vi "helper-RH-create.vi"(7 "Virtual Name":string="_RH", 8 "error in":errorcluster, 9 "record path format OCS\\DB\\%s.* (DISABLE IF EMPTY)":string="OCS\\\\DB\\\\%s.*", 10 "Twet":dbl, 11 "Tdry":dbl) -> (0 "error out":errorcluster, 2 "RH":dbl, 3 "result":string)   [LabVIEW 2024]
uses:
  controls/enumVarCtrlIO.ctl
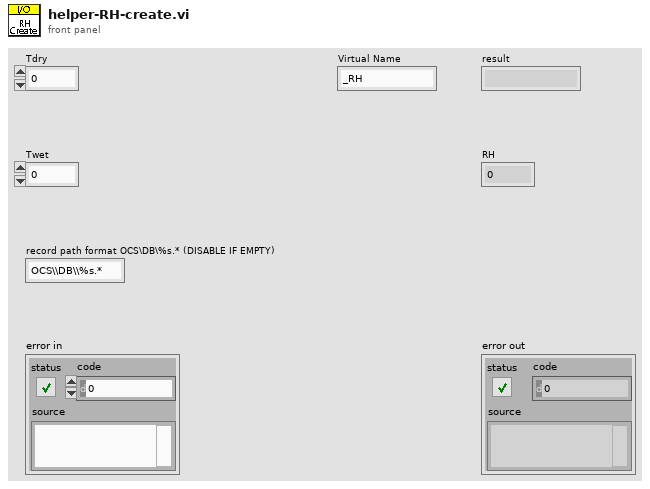
[diagram p1: front panel]
types:
  T1 = typedef "enumVarCtrlIO.ctl" = enum16{"IO Get By Key", "IO List Configs", "IO Add By Key", "IO Modify Value By Key", "IO Modify Calib By Key", "IO Modify ADDR By Key", "IO Modify Mode By Key", "IO Modify Type By Key", "IO Modify Name By Key", "IO Remove By Key", "IO Remove All"}
  T2 = typedef "IONode.ctl" = cluster{"ADDR":T3, "Label":string, "Type":T4, "Mode":T5, "Value":string, "Tags":string, "calibration":T6[]}
  T3 = typedef "type.address.ctl" = u16
  T4 = typedef "enum.io.type.ctl" = enum16{"Type", "DI", "DO", "AI", "AO", "VL", "BUF"}
  T5 = typedef "enum.io.mode.ctl" = enum16{"Mode", "RIO", "SIM"}
  T6 = typedef "typeXyPoint.ctl" = cluster{"X":dbl, "Y":dbl}
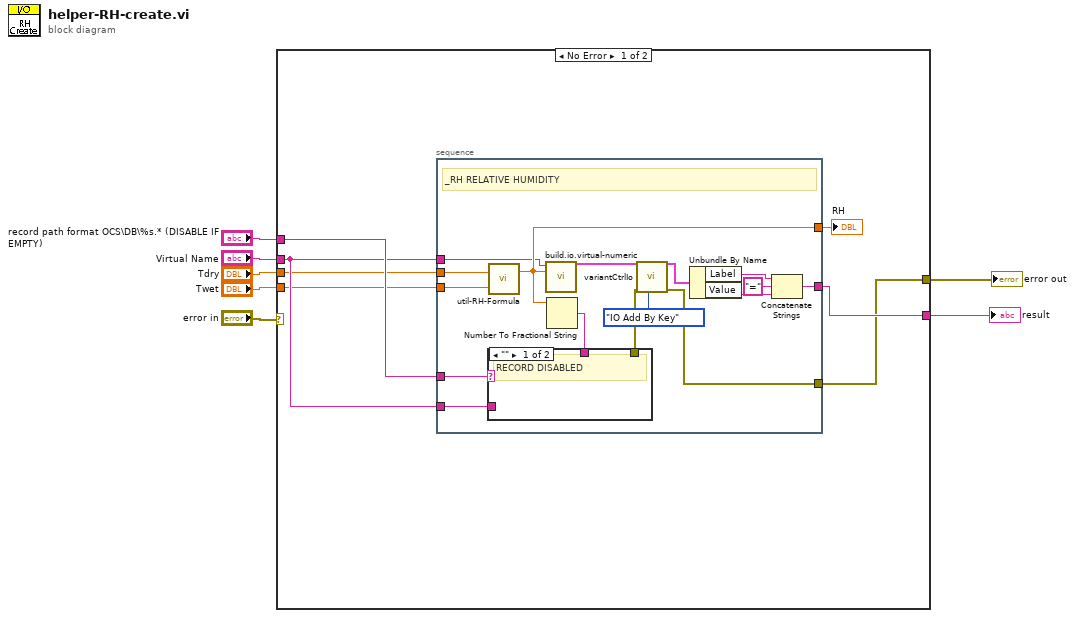
[diagram p0: block diagram]
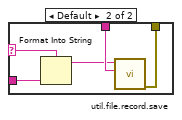
[diagram p2: hidden frame]
diagram:
  n1 = case shown="No Error" "error in" {
    selector: "error in" -> [_ w36]
    tunnel: [w12 w36] -> w7
    tunnel: [w14 _] -> w6
    tunnel: "record path format OCS\\DB\\%s.* (DISABLE IF EMPTY)" -> [w13 _]
    tunnel: "Virtual Name" -> [w11 _]
    tunnel: "Twet" -> [w10 _]
    tunnel: "Tdry" -> [w9 _]
    frame No Error {
      n2 = stacked-sequence {
        tunnel: [w20] -> w8
        tunnel: [w26] -> w12
        tunnel: [w21] -> w14
        tunnel: w13 -> [w15]
        tunnel: w9 -> [w19]
        tunnel: w10 -> [w18]
        tunnel: w11 -> [w17]
        tunnel: w11 -> [w16]
        frame #0 {
          # "_RH RELATIVE HUMIDITY"
          n3 = call "util-RH-Formula.vi"("Twet"=w18, "Tdry"=w19) -> ("RH"=w20:dbl)  [unwired: 1 out]
          n4 = call "build.io.virtual-numeric.vi"("Numeric Value"=w20, "Label"=w17) -> ("IoConf out"=w28:T2)  [unwired: 9 in]
          n5 = Number To Fractional String(number=w20) -> (F-format string=w30:string)  [unwired: 3 in]
          n6 = case shown="\"\"" w15 {
            selector: w15 -> [_ w31]
            tunnel: w30 -> [_ w35]
            tunnel: [_ w34] -> w27
            tunnel: w16 -> [_ w32]
            frame "" {
              # "RECORD DISABLED"
            }
            frame Default {
              n7 = Format Into String(format string=w31, w32) -> (resulting string=w33:string)  [unwired: 2 in, 1 out]
              n8 = call "util.file.record.save.vi"("String Delimited Values"=w35, "record path in"=w33) -> ("error out"=w34:errorcluster)  [unwired: 8 in, 1 out]
            }
          }
          n9 = call "variantCtrlIo.vi"("menu (Get Param)"=enumVarCtrlIO."IO Add By Key" ("menu in (get)"), "error in"=w27, "IOnode in"=w28) -> ("error out"=w26:errorcluster, "IOnode out"=w22:T2)  [unwired: 4 in, 3 out]
          n10 = Unbundle By Name(w22) -> ("Label"=w25:string, "Value"=w24:string)
          n11 = Concatenate Strings(w25, "=" ("string"), w24) -> (w21:string)
        }
      }
      "RH" <- w8
    }
    frame Error {
    }
  }
  "error out" <- w7
  "result" <- w6
